vi "McPherson Setup (VISA).vi"(0 "VISA Resource Name":refnum<visa-resource-name>, 3 "error in":errorcluster, 4 "Action":enum8{"Init McPherson", "Close McPherson"}(ring)) -> (5 "dup VISA Resource Name":refnum<visa-resource-name>, 6 "Setpoint":dbl format="%.2f", 7 "error out":errorcluster)   [LabVIEW 2021]
uses:
  Globals and TypeDefs/Type Definitions.llb/3 way Status.ctl
  Globals and TypeDefs/Error Categories.ctt
  <vilib>/Utility/error.llb/DialogType.ctl
  Serial Instruments/Serial Support VISA.llb/Serial Actions.ctl
  Globals and TypeDefs/gSpectrometer.vi
panel:
  out "X-Axis Unit String":string
  out "UnitFormatString":string="nm"
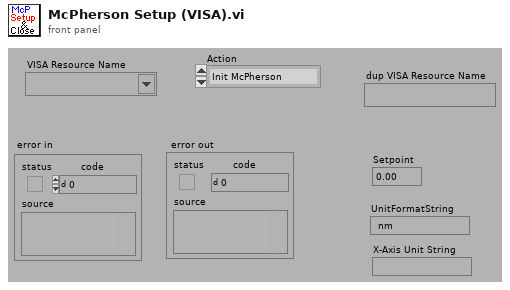
[diagram p1: front panel]
types:
  T1 = typedef "3 way Status.ctl" = u8
  T2 = enum8{"Initialization Error", "Command Error", "Parameter Error", "Overflow Error", "Time-out Error", "Misc Error", "User cancel"}
  T3 = typedef "Error Categories.ctt" = enum8{"General", "CCD-256x1024", "CCD-1340x400", "InGaAs PDA", "McPherson 2075", "Magnetic Field", "Temperature Control", "Other"}
  T4 = typedef "Serial Actions.ctl" = enum16{"Init", "Break", "Clear Buffer", "Write", "Read", "N Bytes", "Lock", "Unlock", "Close"}
  T5 = cluster{"StepperPosition":i32, "MovingStatus":i32, "V":i32, "K":i32, "I":i32}
  T6 = typedef "DialogType.ctl" = u16
  T7 = typedef "McPherson Grating Density.ctl" = enum8{"150", "300", "600", "1200", "1800"}
  T8 = typedef "Wavelength Unit.ctt" = enum8{"Point", "nm", "eV", "meV", "cm_1"}
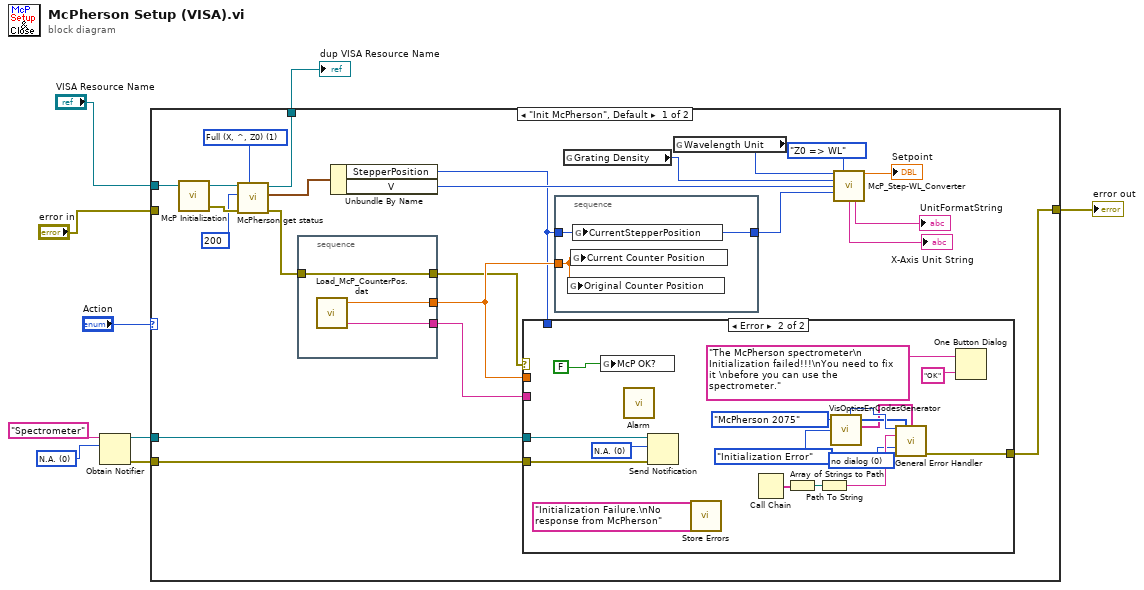
[diagram p0: block diagram]
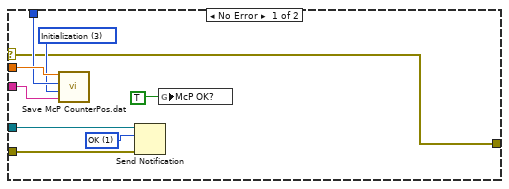
[diagram p2: hidden frame]
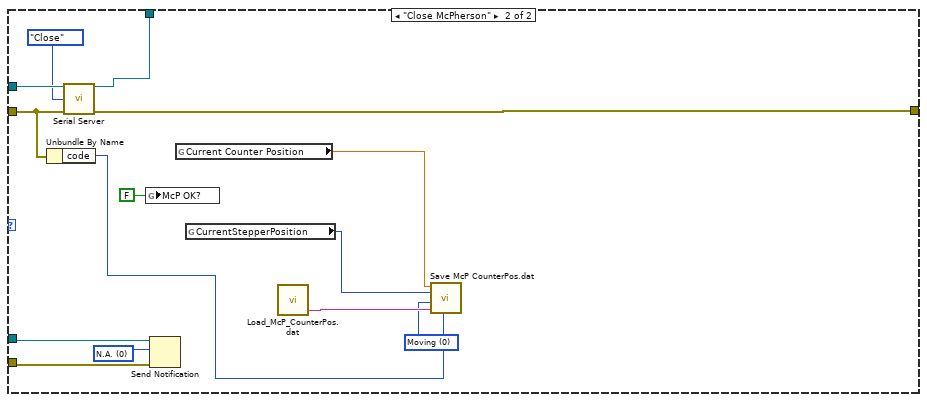
[diagram p3: hidden frame]
diagram:
  w3 = T1 0 items=["N.A.", "OK", "Busy", "Done"] ("Saving")
  n1 = Obtain Notifier(name (unnamed)="Spectrometer", notification data type=w3) -> (notifier out=w2:refnum<notifier>, error out=w1:errorcluster)  [unwired: 2 in, 1 out]
  n2 = case shown="\"Init McPherson\", Default" "Action" {
    tunnel: "VISA Resource Name" -> [w10 w75]
    tunnel: [w22 w73] -> w8
    tunnel: "error in" -> [_ w65]
    tunnel: [w16 w72] -> w6
    tunnel: w2 -> [w18 w67]
    tunnel: w1 -> [w17 w66]
    frame "Init McPherson", Default {
      w24 = u16 1 items=["Grab Globals", "Full (X, ^, Z0)", "Moving(^ and Z0)", "Position(Z0)"] ("Status")
      n3 = call "McP Initialization.vi"("VISA resource name"=w10) -> ("dup VISA Resource Name"=w23:refnum<visa-resource-name>, "error out"=w32:errorcluster)  [unwired: 1 in, 1 out]
      n4 = call "McPherson get status.vi"("Status"=w24, "error in (no error)"=w32, "Wait(ms)"=u32 200, "VISA Resource Name"=w23) -> ("error out"=w31:errorcluster, "StatusParameter"=w14:T5, "dup VISA Resource Name"=w22:refnum<visa-resource-name>)  [unwired: 1 in, 1 out]
      n5 = stacked-sequence {
        tunnel: [w61] -> w19
        tunnel: w31 -> [w61]
        tunnel: [w63] -> w29
        tunnel: [w62] -> w30
        frame #0 {
          n6 = call "Load_McP_CounterPos.dat.VI"() -> ("Counter Position"=w63:dbl, "Last Calibration Date"=w62:string)  [unwired: 1 in, 1 out]
        }
      }
      n7 = Unbundle By Name(w14) -> ("StepperPosition"=w12:i32, "V"=w13:i32)
      n8 = case shown="Error" w19 {
        selector: w19 -> [w35 _]
        tunnel: w30 -> [w43 _]
        tunnel: w29 -> [w42 _]
        tunnel: w12 -> [w41 _]
        tunnel: w18 -> [w36 w56]
        tunnel: w17 -> [w37 w55]
        tunnel: [w35 w44] -> w16
        frame No Error {
          w38 = T1 1 items=["N.A.", "OK", "Busy", "Done"] ("notification")
          w40 = u16 3 items=["Moving", "Calibration", "Key in", "Initialization"] ("Set Method")
          n9 = call "Save McP CounterPos.dat.VI"("Last Calibration Date"=w43, "Set Method"=w40, "McP Stepper Position"=w41, "McP Counter Position"=w42) -> ()  [unwired: 2 in, 1 out]
          n10 = Send Notification(notification=w38, notifier=w36, error in (no error)=w37) -> ()  [unwired: 2 out]
          n11 = global write "gSpectrometer.vi" "McP OK?"(TRUE ("McP OK?")) -> ()
        }
        frame Error {
          w46 = T6 0 items=["no dialog", "OK message", "continue or stop message", "OK message + warnings", "continue/stop + warnings"] ("type of dialog (OK msg:1)")
          w57 = T1 0 items=["N.A.", "OK", "Busy", "Done"] ("notification")
          n12 = global write "gSpectrometer.vi" "McP OK?"(FALSE ("McP OK?")) -> ()
          n13 = call "Alarm.vi"() -> ()  [unwired: 4 in]
          n14 = Send Notification(notification=w57, notifier=w56, error in (no error)=w55) -> ()  [unwired: 2 out]
          n15 = call "Store Errors.vi"("New Error"="Initialization Failure.\nNo response from McPherson") -> ()  [unwired: 1 in]
          n16 = Call Chain() -> (call chain=w52:string[])
          n17 = Array of Strings to Path(0:w52) -> (2:w53:path)  [unwired: 1 in]
          n18 = Path To String(path=w53) -> (string=w54:string)
          n19 = call "VisOpticsErrCodesGenerator.vi"("NHMFL Visible Optics Error Type"=T2."Initialization Error", "NHMFL Visible Optics Error Categories"=Error_Categories.ctt."McPherson 2075") -> ("user-defined descriptions"=w47:string[], "User-defined Error Code"=w51:i32, "user-defined codes"=w48:i32[])  [unwired: 1 in, 3 out]
          n20 = call <vilib>:"General Error Handler.vi"("[error code] (0)"=w51, "[user-defined codes]"=w48, "[user-defined descriptions]"=w47, "[error source] (\" \")"=w54, "type of dialog (OK msg:1)"=w46) -> ("error out"=w44:errorcluster)  [unwired: 6 in, 4 out]
          n21 = One Button Dialog(message="The McPherson spectrometer\n Initialization failed!!!\nYou need to fix it \nbefore you can use the spectrometer.", button name ("OK")="OK") -> ()  [unwired: 1 out]
        }
      }
      n22 = stacked-sequence {
        tunnel: w29 -> [w34]
        tunnel: [w33] -> w25
        tunnel: w12 -> [w33]
        frame #0 {
          n23 = global write "gSpectrometer.vi" "Original Counter Position"(w34) -> ()
          n24 = global write "gSpectrometer.vi" "Current Counter Position"(w34) -> ()
          n25 = global write "gSpectrometer.vi" "CurrentStepperPosition"(w33) -> ()
        }
      }
      n26 = global read "gSpectrometer.vi" "Grating Density"() -> (w21:T7)
      n27 = global read "gSpectrometer.vi" "Wavelength Unit"() -> (w20:T8)
      n28 = call "McP_Step-WL_Converter.vi"("Wavelength Unit"=w20, "Option (Z0 <=> WL)"=enum16{"Z0 => WL", "WL => Z0", "Update WL only"}."Z0 => WL", "Grating Density"=w21, "Velocity (Steps/s)"=w13, "Stepper Position Input"=w25) -> ("Wavelength Output"=→"Setpoint":dbl, "X-Axis Unit String"=→"X-Axis Unit String":string, "UnitFormatString"=→"UnitFormatString":string)  [unwired: 3 in, 5 out]
    }
    frame "Close McPherson" {
      w68 = T1 0 items=["N.A.", "OK", "Busy", "Done"] ("notification")
      w76 = u16 0 items=["Moving", "Calibration", "Key in", "Initialization"] ("Set Method")
      n29 = Unbundle By Name(w65) -> ("code"=w64:i32)
      n30 = call "Serial Server.vi"("VISA Resource Name"=w75, "Action"=Serial_Actions."Close", "error in (no error)"=w65) -> ("dup VISA Resource Name"=w73:refnum<visa-resource-name>, "error out"=w72:errorcluster)  [unwired: 8 in, 3 out]
      n31 = global write "gSpectrometer.vi" "McP OK?"(FALSE ("McP OK?")) -> ()
      n32 = Send Notification(notification=w68, notifier=w67, error in (no error)=w66) -> ()  [unwired: 2 out]
      n33 = global read "gSpectrometer.vi" "Current Counter Position"() -> (w70:dbl)
      n34 = global read "gSpectrometer.vi" "CurrentStepperPosition"() -> (w69:i32)
      n35 = call "Load_McP_CounterPos.dat.VI"() -> ("Last Calibration Date"=w77:string)  [unwired: 1 in, 2 out]
      n36 = call "Save McP CounterPos.dat.VI"("Error Code (0: No Error)"=w64, "Last Calibration Date"=w77, "Set Method"=w76, "McP Stepper Position"=w69, "McP Counter Position"=w70) -> ()  [unwired: 1 in, 1 out]
    }
  }
  "dup VISA Resource Name" <- w8
  "error out" <- w6
